vi "Normalized to Encoder Velocity.vi"(8 "Enum":enum16{"JV", "Mule", "Linda/Sophie"}(ring), 11 "ft/s":dbl) -> (3 "Output":dbl)   [LabVIEW 2019]
doc: "Converting from ft/s to Rev/min (for sparks) or ticks/100ms (for Talons)"
panel:
  in  "y 2":dbl=11.0
  in  "y":dbl=0.85 format="%#_13g"
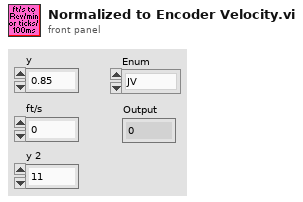
[diagram p1: front panel]
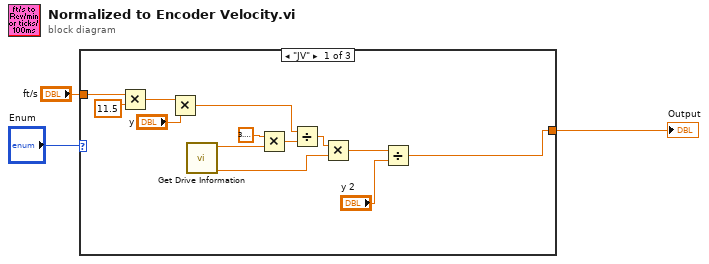
[diagram p0: block diagram]
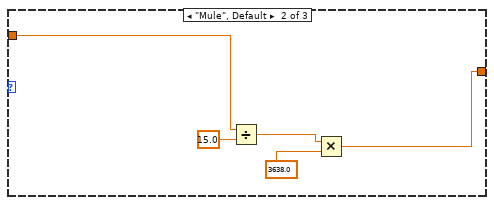
[diagram p2: hidden frame]
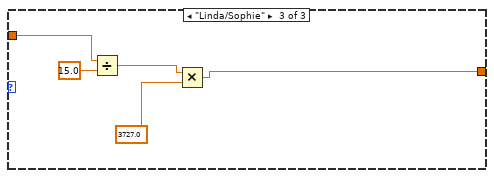
[diagram p3: hidden frame]
diagram:
  n1 = case shown="\"JV\"" "Enum" {
    tunnel: "ft/s" -> [w16 w19 w26]
    tunnel: [w5 w18 w22] -> w1
    frame "JV" {
      n2 = Multiply(x=w16, y=11.5) -> (x*y=w8:dbl)
      n3 = Multiply(x=w8, y="y") -> (x*y=w6:dbl)
      n4 = call "Get Drive Information.vi"() -> ("Ticks/Revolution"=w9:dbl, "Wheel Diameter"=w10:dbl)  [unwired: 10 in]
      n5 = Multiply(x=3.141592653589793, y=w10) -> (x*y=w13:dbl)
      n6 = Divide(x=w6, y=w13) -> (x/y=w12:dbl)
      n7 = Multiply(x=w12, y=w9) -> (x*y=w11:dbl)
      n8 = Divide(x=w11, y="y 2") -> (x/y=w5:dbl)
    }
    frame "Mule", Default {
      n9 = Divide(x=w19, y=15.0) -> (x/y=w20:dbl)
      n10 = Multiply(x=w20, y=3638.0 ("y 2")) -> (x*y=w18:dbl)
    }
    frame "Linda/Sophie" {
      n11 = Divide(x=w26, y=15.0) -> (x/y=w24:dbl)
      n12 = Multiply(x=w24, y=3727.0 ("Scaling")) -> (x*y=w22:dbl)
    }
  }
  "Output" <- w1
